vi "NI VeriStand - Advanced Browsing Dialog.vi"(5 "Pattern Label":string, 6 "File Pattern":string, 7 "CtlRef":refnum<vi>, 8 "error in (no error)":errorcluster, 9 "Most recent path":path, 10 "Paths":path[](array[path]), 11 "Dialog Title":string) -> (0 "error out":errorcluster, 2 "Most recent folder":path, 3 "Selected file":path, 4 "Valid?":bool)   [LabVIEW 2020, in "Custom Device Utility Library.lvlib"]
doc: "Configures an advanced browsing dialog box for files that match the <B>File Pattern</B> you specify. This VI creates the same style browsing dialog that appears in NI VeriStand if you select <B>Advanced browsing</B> on the <B>Folder Start Paths</B> page of the <B>Options</B> dialog box."
uses:
  <vilib>/NI VeriStand/Custom Device Tools/Custom Device Utility Library/Custom Device Utility Library.lvlib
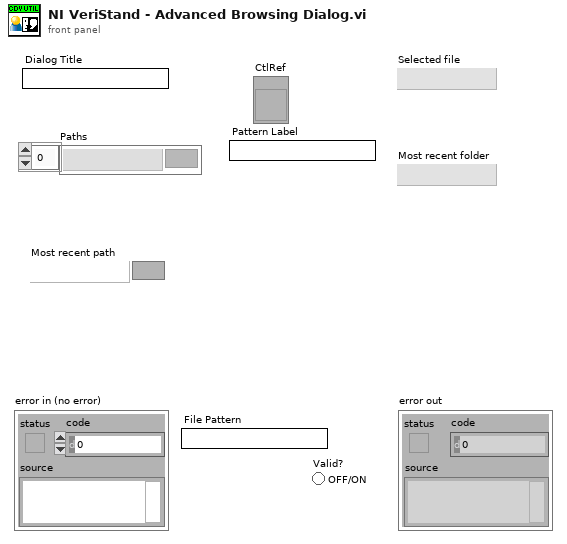
[diagram p1: front panel]
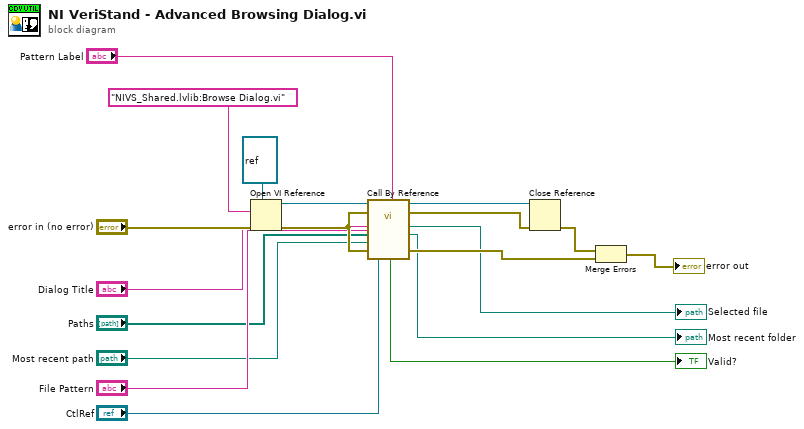
[diagram p0: block diagram]
diagram:
  n1 = Open VI Reference(type specifier VI Refnum (for type only)=refnum<vi> refnum, vi path="NIVS_Shared.lvlib:Browse Dialog.vi", error in (no error)="error in (no error)") -> (vi reference=w11:refnum<vi>, error out=w10:errorcluster)  [unwired: 3 out]
  n2 = call-by-ref "?"(reference=w11, error in=w10, "Pattern Label"="Pattern Label", "CtlRef"="CtlRef", "Pattern"="File Pattern", 8:"error in (no error)"=w10, "Most recent path"="Most recent path", "Paths"="Paths", "Title (\"\" Default title)"="Dialog Title") -> (reference out=w16:refnum<vi>, error out=w17:errorcluster, 0:"error out"=w18:errorcluster, "Most recent folder"=→"Most recent folder":path, "Selected file"=→"Selected file":path, "Valid?"=→"Valid?":bool)  [unwired: 1 in]
  n3 = Close Reference(reference=w16, error in (no error)=w17) -> (error out=w15:errorcluster)
  n4 = Merge Errors(w15, w18) -> (→"error out":errorcluster)
